vi "lab3_sim_channel_coding_v3.vi"() -> ()   [LabVIEW 2014]
uses:
  <vilib>/addons/Modulation/Digital/General/MT Generate Bits (Galois, PN Order).vi
  <vilib>/addons/Modulation/Digital/Support/Common/Validators/mod_Generate Bits Validate.vi
  <vilib>/addons/Modulation/Analog/support/mod_Set Error Source.vi
  <vilib>/addons/Modulation/Digital/General/subVIs/mod_Generate Bits PN Sequence.vi
  <vilib>/addons/Modulation/niDMT.lvlib
  <vilib>/Analysis/NI_AALBase.lvlib
panel:
  out "Constellation Graph":cdb[](graph)
  out "Error bits":i16
  out "Decoded":bool[](array[boolean])
  out "output in decimal":u32[][](array[numeric])
  out "state transition":u32[][](array[numeric])
  out "coded bits":i16[](array[numeric])
  in  "decision type":enum16{"hard decision", "soft decision"}(ring)
  in  "Tab Control":T1(tab)
  in  "modulation 2":enum16{"BPSK", "QPSK"}(ring)
  in  "modulation 3":enum16{"BPSK", "QPSK"}(ring)
  in  "modulation":enum16{"BPSK", "QPSK", "16QAM"}(ring)
  out "message":bool[](array[boolean])
  in  "Eb/N0 (dB)":dbl
  in  "stop":bool
  in  "total message bits":i32=128
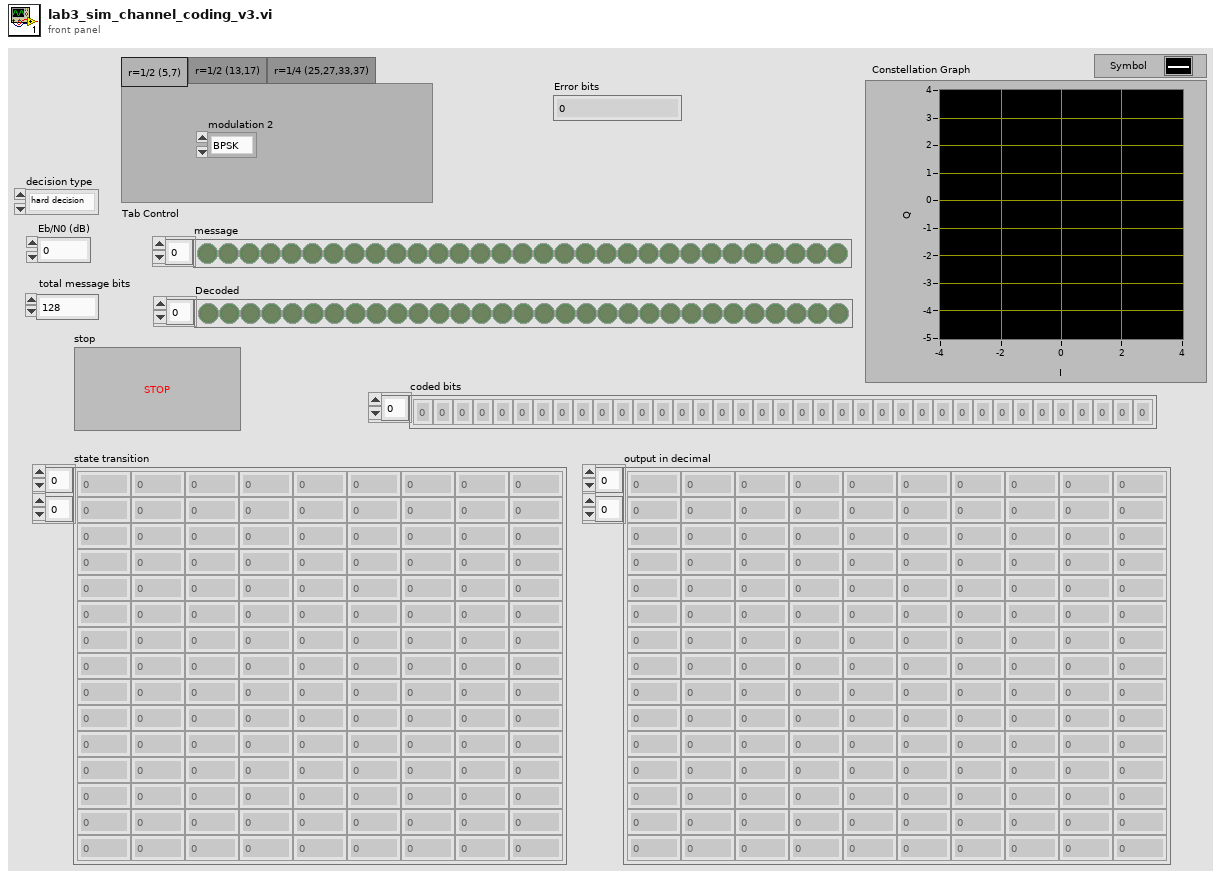
[diagram p1: front panel]
types:
  T1 = enum32{"r=1/2 (5,7)", "r=1/2 (13,17)", "r=1/4 (25,27,33,37)"}
  T2 = enum16{"r=1/2 (5,7)", "r=1/2 (13,17)", "r=1/4 (25,27,33,37)"}
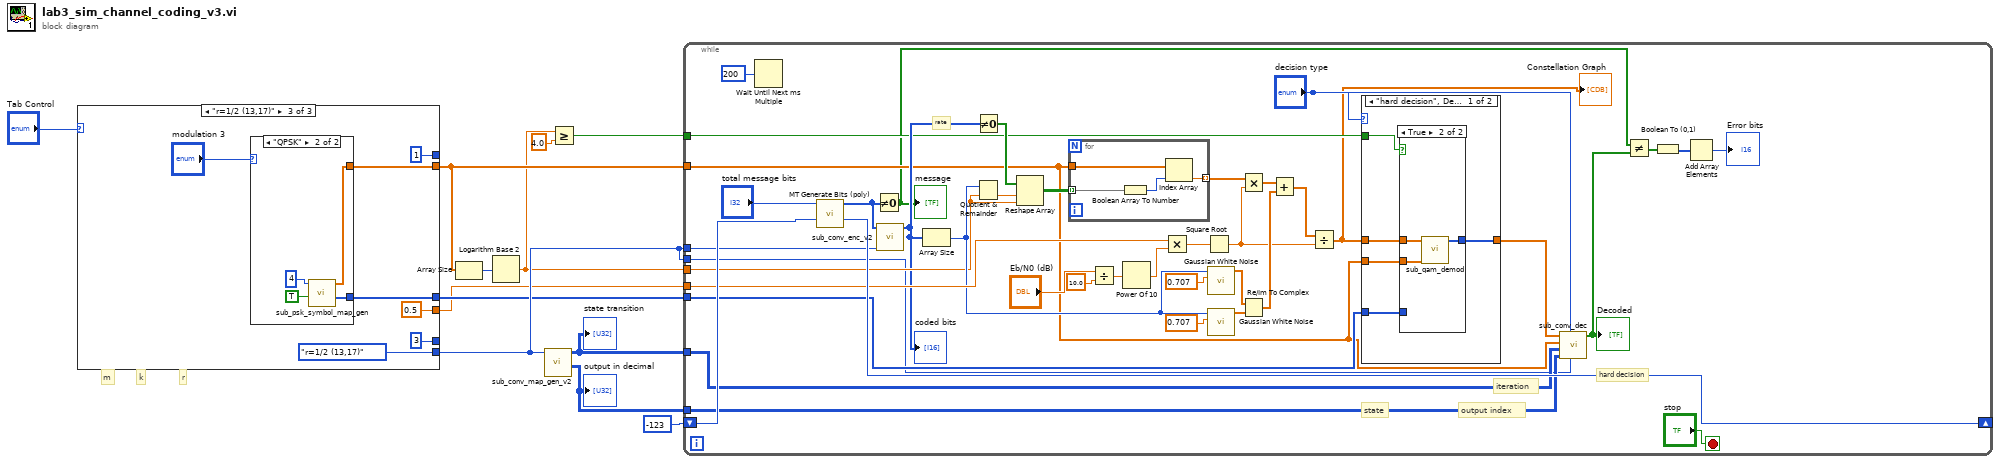
[diagram p0: block diagram]
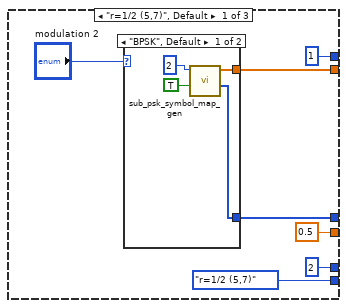
[diagram p2: hidden frame]
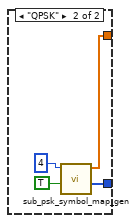
[diagram p3: hidden frame]
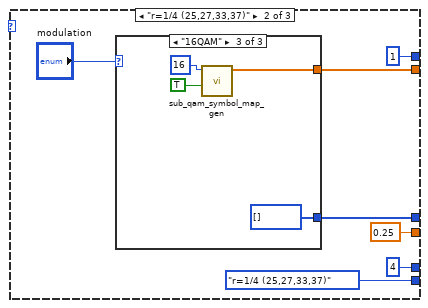
[diagram p4: hidden frame]
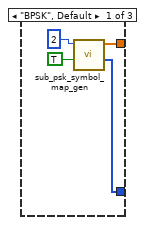
[diagram p5: hidden frame]
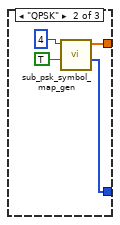
[diagram p6: hidden frame]
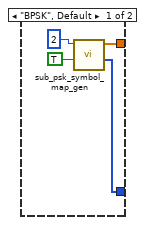
[diagram p7: hidden frame]
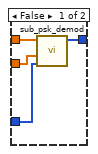
[diagram p8: hidden frame]
diagram:
  # "r"
  # "m"
  # "k"
  n1 = case shown="\"r=1/2 (13,17)\"" "Tab Control" {
    tunnel: [T2."r=1/2 (5,7)" ("code type") T2."r=1/4 (25,27,33,37)" ("code type") T2."r=1/2 (13,17)" ("code type")] -> w6
    tunnel: [w17 w32 w51] -> w9
    tunnel: [1 1 1] -> _
    tunnel: [2 4 3] -> _
    tunnel: [0.5 0.25 0.5] -> w1
    tunnel: [w13 w28 w47] -> w2
    frame "r=1/2 (5,7)", Default {
      n2 = case shown="\"BPSK\", Default" "modulation 2" {
        tunnel: [w23 w27] -> w17
        tunnel: [w22 w26] -> w13
        frame "BPSK", Default {
          n3 = call "sub_psk_symbol_map_gen.vi"("Gray code?"=TRUE, "M-PSK"=2) -> ("index map"=w22:u32[], "symbol map"=w23:cdb[])  [unwired: 8 in]
        }
        frame "QPSK" {
          n4 = call "sub_psk_symbol_map_gen.vi"("Gray code?"=TRUE, "M-PSK"=4) -> ("index map"=w26:u32[], "symbol map"=w27:cdb[])  [unwired: 8 in]
        }
      }
    }
    frame "r=1/4 (25,27,33,37)" {
      n5 = case shown="\"16QAM\"" "modulation" {
        tunnel: [w38 w42 w46] -> w32
        tunnel: [w37 w41 u32[] [] ("index map")] -> w28
        frame "BPSK", Default {
          n6 = call "sub_psk_symbol_map_gen.vi"("Gray code?"=TRUE, "M-PSK"=2) -> ("index map"=w37:u32[], "symbol map"=w38:cdb[])  [unwired: 8 in]
        }
        frame "QPSK" {
          n7 = call "sub_psk_symbol_map_gen.vi"("Gray code?"=TRUE, "M-PSK"=4) -> ("index map"=w41:u32[], "symbol map"=w42:cdb[])  [unwired: 8 in]
        }
        frame "16QAM" {
          n8 = call "sub_qam_symbol_map_gen.vi"("Gray code?"=TRUE, "M-QAM"=16) -> ("symbol map"=w46:cdb[])  [unwired: 9 in]
        }
      }
    }
    frame "r=1/2 (13,17)" {
      n9 = case shown="\"QPSK\"" "modulation 3" {
        tunnel: [w57 w61] -> w51
        tunnel: [w56 w60] -> w47
        frame "BPSK", Default {
          n10 = call "sub_psk_symbol_map_gen.vi"("Gray code?"=TRUE, "M-PSK"=2) -> ("index map"=w56:u32[], "symbol map"=w57:cdb[])  [unwired: 8 in]
        }
        frame "QPSK" {
          n11 = call "sub_psk_symbol_map_gen.vi"("Gray code?"=TRUE, "M-PSK"=4) -> ("index map"=w60:u32[], "symbol map"=w61:cdb[])  [unwired: 8 in]
        }
      }
    }
  }
  n12 = Array Size(array=w9) -> (size(s)=w10:i32)
  n13 = Logarithm Base 2(1:w10) -> (0:w5:dbl)
  n14 = call "sub_conv_map_gen_v2.vi"("code type"=w6) -> ("output in decimal"=w7:u32[][], "state transition"=w8:u32[][])  [unwired: 9 in]
  "state transition" <- w8
  "output in decimal" <- w7
  n15 = Greater Or Equal?(x=w5, y=4.0) -> (x >= y?=w3:bool)
  n16 = while {
    shift-right: [w102] -> _
    shift-left: -123 ("seed out") -> [w103]
    tunnel: w1 -> [w86]
    tunnel: w5 -> [w79]
    tunnel: w9 -> [w71]
    tunnel: w6 -> [w68]
    tunnel: w8 -> [w70]
    tunnel: w7 -> [w69]
    tunnel: w6 -> [w76]
    tunnel: w3 -> [w75]
    tunnel: w2 -> [w74]
    stop <- "stop" stop-if-true
    # "output index"
    # "state"
    # "iteration"
    # "hard decision"
    # "rate"
    n17 = Wait Until Next ms Multiple(millisecond multiple=u32 200) -> ()  [unwired: 1 out]
    n18 = call-poly <vilib>:"MT Generate Bits (poly).vi"("total bits (128)"="total message bits", "seed in (0xD6BF7DF2)"=w103) -> ("output bit stream"=w77:i8[], "seed out"=w102:i32)  [unwired: 11 in, 1 out]
    n19 = Not Equal To 0?(x=w77) -> (x != 0?=w67:bool[])
    "message" <- w67
    n20 = call "sub_conv_enc_v2.vi"("code type"=w76, "bitstream"=w77) -> ("coded bits"=w78:i16[])  [unwired: 9 in]
    "coded bits" <- w78
    n21 = Array Size(array=w78) -> (size(s)=w83:i32)
    n22 = Not Equal To 0?(x=w78) -> (x != 0?=w84:bool[])
    n23 = Quotient & Remainder(x=w83, y=w79) -> (floor(x/y)=w82:dbl)  [unwired: 1 out]
    n24 = Reshape Array(w84, w82, w79) -> (w81:bool[][])
    n25 = for {
      tunnel: w81 -> [w120] mode=indexing
      tunnel: w71 -> [w119]
      tunnel: [w117] -> w80 mode=indexing
      n26 = Boolean Array To Number(Boolean array=w120) -> (number=w118:u32)
      n27 = Index Array(array=w119, index=w118) -> (element=w117:cdb)
    }
    n28 = Divide(x="Eb/N0 (dB)", y=10.0) -> (x/y=w97:dbl)
    n29 = Power Of 10(x=w97) -> (10^x=w87:dbl)
    n30 = Multiply(x=w86, y=w87) -> (x*y=w85:dbl)
    n31 = Square Root(x=w85) -> (sqrt(x)=w90:dbl)
    n32 = call <vilib>:"Gaussian White Noise.vi"("standard deviation"=0.707, "samples"=w83) -> ("Gaussian noise pattern"=w94:dbl[])  [unwired: 8 in, 1 out]
    n33 = call <vilib>:"Gaussian White Noise.vi"("standard deviation"=0.707, "samples"=w83) -> ("Gaussian noise pattern"=w93:dbl[])  [unwired: 8 in, 1 out]
    n34 = Multiply(x=w80, y=w90) -> (x*y=w92:cdb[])
    n35 = Re/Im To Complex(1:w93, 2:w94) -> (0:w91:cdb[])
    n36 = Add(x=w92, y=w91) -> (x+y=w89:cdb[])
    n37 = Divide(x=w89, y=w90) -> (x/y=w62:cdb[])
    "Constellation Graph" <- w62
    n38 = case shown="\"hard decision\", Default" "decision type" {
      tunnel: w62 -> [w107 w116]
      tunnel: w75 -> [w108 _]
      tunnel: w71 -> [w106 _]
      tunnel: w74 -> [w105 _]
      tunnel: [w104 w116] -> w73
      frame "hard decision", Default {
        n39 = case shown="True" w108 {
          tunnel: w107 -> [w112 w115]
          tunnel: w106 -> [w111 w114]
          tunnel: [w109 w113] -> w104
          tunnel: w105 -> [w110 _]
          frame False {
            n40 = call "sub_psk_demod.vi"("index map"=w110, "symbol map"=w111, "symbol"=w112) -> ("bitstream"=w109:i16[])  [unwired: 8 in]
          }
          frame True {
            n41 = call "sub_qam_demod.vi"("symbol map"=w114, "symbol"=w115) -> ("bitstream"=w113:i16[])  [unwired: 9 in]
          }
        }
      }
      frame "soft decision" {
      }
    }
    n42 = call "sub_conv_dec.vi"("code type"=w68, "decision type"="decision type", "output in decimal"=w69, "state transition"=w70, "symbol map"=w71, "hard bits/soft symbols"=w73) -> ("Decoded"=w66:bool[])  [unwired: 5 in]
    "Decoded" <- w66
    n43 = Not Equal?(x=w67, y=w66) -> (x != y?=w65:bool[])
    n44 = Boolean To (0,1)(Boolean=w65) -> (0, 1=w64:i16[])
    n45 = Add Array Elements(numeric array=w64) -> (sum=→"Error bits":i16)
  }
